vi "Set Number Prog.vi"(8 "error in (no error)":errorcluster caption="entrée d'erreur (pas d'erreur)", 10 "Number Prog":string, 11 "Class Camera Pattern Matching (Default) en entrée":refnum<class "Class Pattern Matching (Default).lvclass">) -> (0 "error out":errorcluster caption="sortie d'erreur", 3 "Class Camera Pattern Matching (Default) en sortie":refnum<class "Class Pattern Matching (Default).lvclass">)   [LabVIEW 2020, in "Library Instrument & Equipement.lvlib" / "Library Camera.lvlib" / "Class Pattern Matching (Default).lvclass"]
uses:
  Class Pattern Matching (Default).lvclass
  Class Pattern Matching (Default).lvclass/Class Pattern Matching (Default).ctl
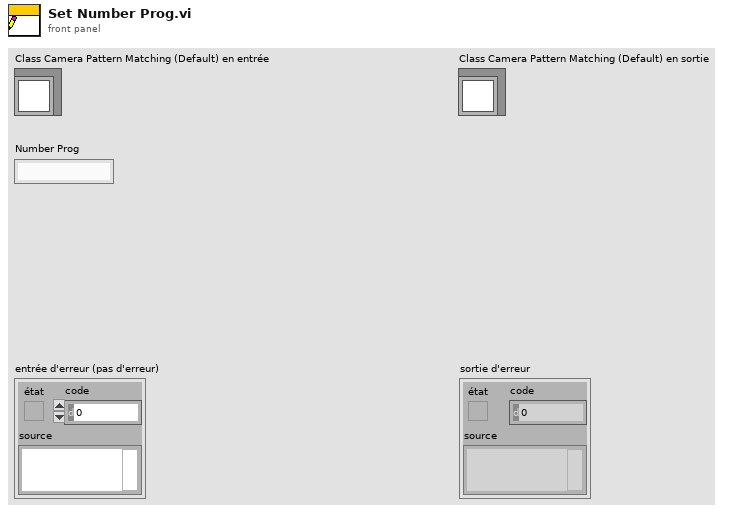
[diagram p1: front panel]
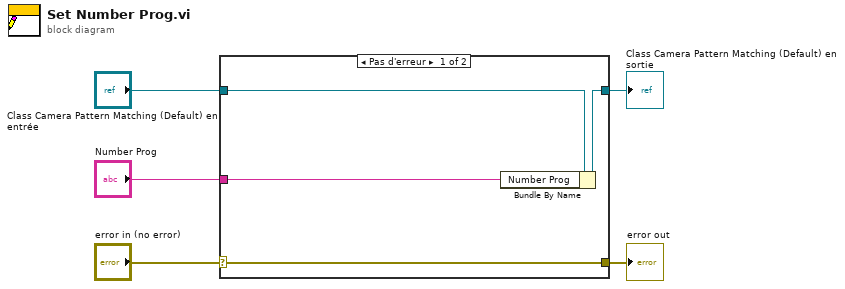
[diagram p0: block diagram]
diagram:
  n1 = case shown="Pas d'erreur" "error in (no error)" {
    selector: "error in (no error)" -> [w9 w10]
    tunnel: [w9 w10] -> w4
    tunnel: [w7 w11] -> w2
    tunnel: "Class Camera Pattern Matching (Default) en entrée" -> [w8 w11]
    tunnel: "Number Prog" -> [w6 _]
    frame No Error {
      n2 = Bundle By Name(cluster=w8, "Number Prog"=w6) -> (w7:refnum<class "Class Pattern Matching (Default).lvclass">)
    }
    frame Error {
    }
  }
  "error out" <- w4
  "Class Camera Pattern Matching (Default) en sortie" <- w2
